vi "Unix epoch time to timestamp.vi"(10 "Precision (ms)":T1=enum."milliseconds", 11 "Unix epoch time":u64) -> (3 "Time Stamp":timestamp format="%<%I:%M:%S%3u %p\n%Y/%m/%d>T")   [LabVIEW 2013, in "InfluxDB Client.lvclass"]
doc: "Convert Unix epoch time to the LabVIEW timestamp format."
uses:
  InfluxDB Client.lvclass
  Time precision.ctl
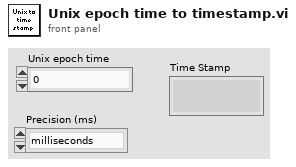
[diagram p1: front panel]
types:
  T1 = typedef "InfluxDB Client.lvclass/Time precision.ctl" = enum16{"seconds", "milliseconds", "microseconds"}
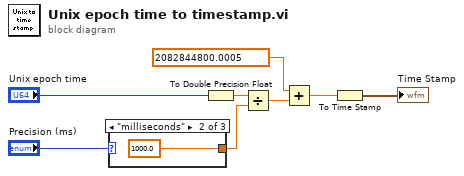
[diagram p0: block diagram]
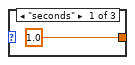
[diagram p2: hidden frame]
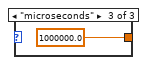
[diagram p3: hidden frame]
diagram:
  n1 = case shown="\"milliseconds\"" "Precision (ms)" {
    tunnel: [1.0 ("Database name") 1000.0 ("Database name") 1000000.0 ("Database name")] -> w5
    frame "seconds" {
    }
    frame "milliseconds" {
    }
    frame "microseconds" {
    }
  }
  n2 = To Double Precision Float(number="Unix epoch time") -> (double precision float=w6:dbl)
  n3 = Divide(x=w6, y=w5) -> (x/y=w3:dbl)
  n4 = Add(x=2082844800.0005, y=w3) -> (x+y=w2:dbl)
  n5 = To Time Stamp(1:w2) -> (0:→"Time Stamp":timestamp)
